vi "fir_test2.vi"() -> ()   [LabVIEW 2013]
uses:
  <vilib>/Analysis/NI_AALBase.lvlib
panel:
  out "Max Generated":dbl
  out "Simulated":dbl[][](graph)
  in  "stop":bool
  out "Filtered":dbl(graph)
  out "Max":fxp<+/-,16,16>
  out "rdy":bool
  out "# of Iterations":i32
  out "data_valid":bool
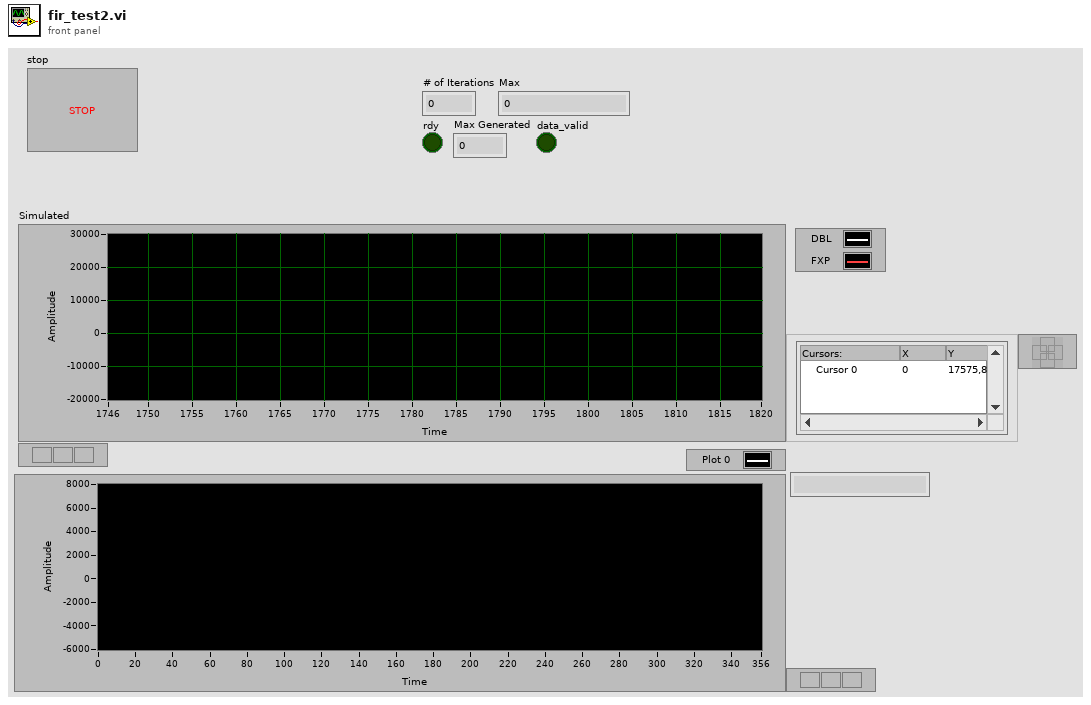
[diagram p1: front panel]
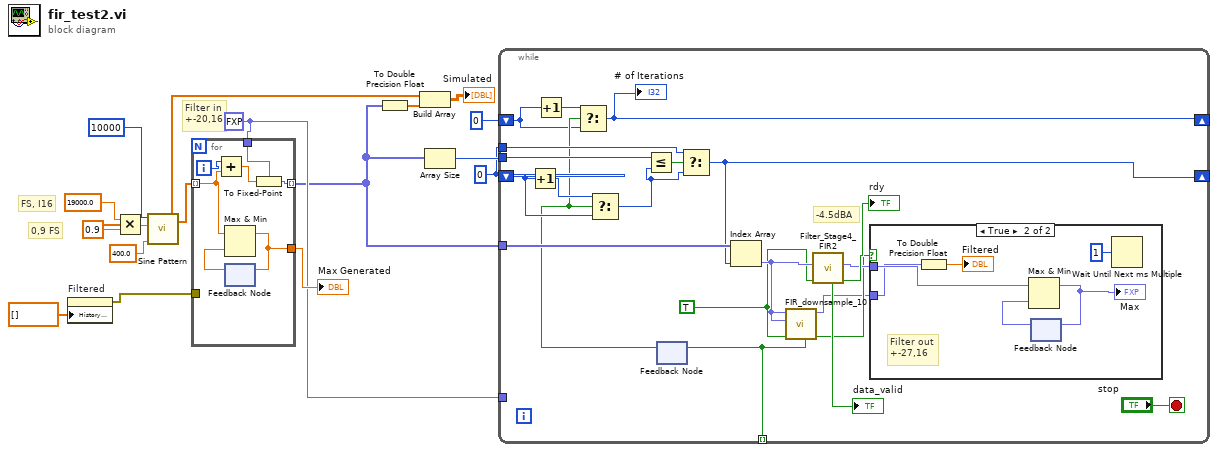
[diagram p0: block diagram]
diagram:
  w3 = fxp<+/-,25,19> 0.0 ("fixed-point type")
  w11 = 0 ("samples")
  # "Filter in\n+-20,16"
  # "FS, I16"
  # "0,9 FS"
  n1 = property on="Filtered" class="WFChart (strict)"("History Data"=dbl[] []) -> (error out=w5:errorcluster)  [unwired: 2 in, 1 out]
  n2 = Multiply(x=19000.0 ("amplitude"), y=0.9) -> (x*y=w13:dbl)
  n3 = call <vilib>:"Sine Pattern.vi"("cycles"=400.0, "amplitude"=w13, "samples"=10000) -> ("Sinusoidal Pattern"=w9:dbl[])  [unwired: 1 in, 1 out]
  n4 = for {
    tunnel: w9 -> [w19] mode=indexing
    tunnel: [w23] -> w1 mode=indexing
    tunnel: w3 -> [w22]
    tunnel: [w20] -> w6
    tunnel: w5 -> [_]
    i -> [w18]
    n5 = Add(x=w18, y=w19) -> (x+y=w17:dbl)
    n6 = feedback #1() -> (w21:dbl)  [unwired: 1 in]
    n7 = Max & Min(x=w19, y=w21) -> (max(x,y)=w20:dbl)  [unwired: 1 out]
    n8 = feedback-in #1(w20) -> ()
    n9 = To Fixed-Point(fixed-point type=w22, number=w17) -> (fixed-point=w23:fxp<+/-,25,19>)
  }
  "Max Generated" <- w6
  n10 = To Double Precision Float(number=w1) -> (double precision float=w10:dbl[])
  n11 = Build Array(w9, w10) -> (→"Simulated":dbl[][])
  n12 = Array Size(array=w1) -> (size(s)=w12:i32)
  n13 = while {
    tunnel: w1 -> [w42]
    shift-right: [w41] -> _
    shift-left: w11 -> [w30]
    tunnel: w12 -> [w40]
    tunnel: w11 -> [w43]
    tunnel: w3 -> [_]
    shift-right: [w26] -> _
    shift-left: 0 ("samples") -> [w25]
    tunnel: [w24] -> _ mode=indexing
    stop <- "stop" stop-if-true
    w33 = TRUE
    # "-4.5dBA"
    n14 = Increment(x=w30) -> (x+1=w31:i32)
    n15 = Increment(x=w25) -> (x+1=w27:i32)
    n16 = feedback #2() -> (w28:bool)  [unwired: 1 in]
    n17 = Select(t=w27, s=w28, f=w25) -> (s? t:f=w26:i32)
    "# of Iterations" <- w26
    n18 = Select(t=w31, s=w28, f=w30) -> (s? t:f=w29:i32)
    n19 = Less Or Equal?(x=w40, y=w29) -> (x <= y?=w37:bool)
    n20 = Select(t=w43, s=w37, f=w29) -> (s? t:f=w41:i32)
    n21 = Index Array(array=w42, index=w41) -> (element=w35:fxp<+/-,25,19>)
    n22 = call "FIR_downsample_10.vi"("valid in"=w33, "Q in"=w35, "I in"=w35) -> ("valid out"=w34:bool, "I out"=w32:fxp<+/-,16,16>, "ready for input"=w24:bool)  [unwired: 5 in, 1 out]
    n23 = feedback-in #2(w24) -> ()
    n24 = call "Filter_Stage4_FIR2.vi"("nd"=w33, "I in"=w35) -> ("rdy"=→"rdy":bool, "I out"=w38:fxp<+/-,16,16>, "data_valid"=→"data_valid":bool)  [unwired: 4 in, 3 out]
    n25 = case shown="True" w34 {
      tunnel: w38 -> [_ w46]
      tunnel: w32 -> [_ w45]
      frame False {
      }
      frame True {
        # "Filter out\n+-27,16"
        n26 = To Double Precision Float(number=w45) -> (double precision float=→"Filtered":dbl)
        n27 = feedback #3() -> (w49:fxp<+/-,16,16>)  [unwired: 1 in]
        n28 = Max & Min(x=w46, y=w49) -> (max(x,y)=w48:fxp<+/-,16,16>)  [unwired: 1 out]
        "Max" <- w48
        n29 = feedback-in #3(w48) -> ()
        n30 = Wait Until Next ms Multiple(millisecond multiple=u32 1) -> ()  [unwired: 1 out]
      }
    }
  }
